vi "Add post to experiment.vi"(7 "API Key":string, 8 "error in":errorcluster, 10 "Thread ID":i32, 11 "Post contents":string) -> (0 "error out":errorcluster)   [LabVIEW 2018]
uses:
  <vilib>/httpClient/POSTBuffer.vi
  <vilib>/httpClient/LabVIEWHTTPClient.lvlib
panel:
  out "Comment ID":i32
  out "Server response debug panel":string
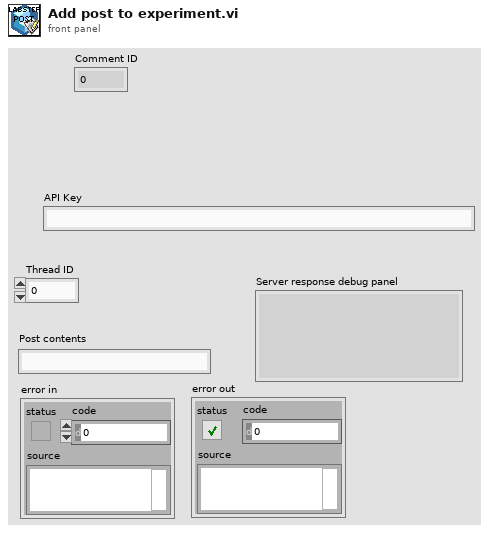
[diagram p1: front panel]
types:
  T1 = typedef "LabVIEWHTTPClient.lvlib/ClientHandle.ctl" = refnum<k1>
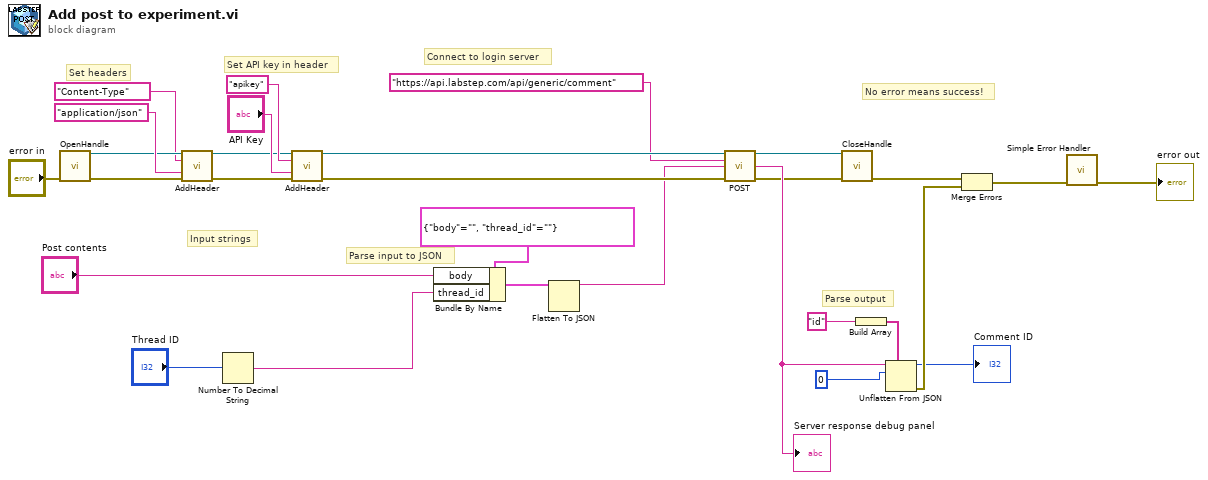
[diagram p0: block diagram]
diagram:
  # "No error means success!"
  # "Parse output"
  # "Set API key in header"
  # "Input strings"
  # "Set headers"
  # "Connect to login server"
  # "Parse input to JSON"
  n1 = call <vilib>:"OpenHandle.vi"("error in (no error)"="error in") -> ("client handle out"=w28:T1, "error out"=w27:errorcluster)  [unwired: 13 in]
  n2 = call <vilib>:"AddHeader.vi"("client handle"=w28, "header"="Content-Type", "value"="application/json", "error in (no error)"=w27) -> ("client handle out"=w17:T1, "error out"=w20:errorcluster)  [unwired: 10 in]
  n3 = Number To Decimal String(number="Thread ID") -> (decimal integer string=w4:string)  [unwired: 1 in]
  n4 = call <vilib>:"AddHeader.vi"("client handle"=w17, "header"="apikey", "value"="API Key", "error in (no error)"=w20) -> ("client handle out"=w18:T1, "error out"=w19:errorcluster)  [unwired: 10 in]
  n5 = Bundle By Name(cluster=cluster{"body":string, "thread_id":string} {"body"="", "thread_id"=""}, "body"="Post contents", "thread_id"=w4) -> (w26:cluster{"body":string, "thread_id":string})
  n6 = Flatten To JSON(anything=w26) -> (JSON string=w16:string)  [unwired: 2 in, 1 out]
  n7 = call-poly <vilib>:"POST.vi"("client handle"=w18, "url"="https://api.labstep.com/api/generic/comment", "buffer"=w16, "error in (no error)"=w19) -> ("client handle out"=w11:T1, "body"=w13:string, "error out"=w10:errorcluster)  [unwired: 8 in, 1 out]
  "Server response debug panel" <- w13
  n8 = call <vilib>:"CloseHandle.vi"("client handle"=w11, "error in (no error)"=w10) -> ("error out"=w8:errorcluster)  [unwired: 13 in]
  n9 = Build Array("id") -> (w14:string[])
  n10 = Unflatten From JSON(path=w14, JSON string=w13, type and defaults=0) -> (value=→"Comment ID":i32, error out=w7:errorcluster)  [unwired: 4 in]
  n11 = Merge Errors(w8, w7) -> (w12:errorcluster)
  n12 = call <vilib>:"Simple Error Handler.vi"("error in (no error)"=w12) -> ("error out"=→"error out":errorcluster)  [unwired: 4 in, 4 out]
